vi "Min_Max_Entry.vi"() -> ()   [LabVIEW 2019]
uses:
  Global Variables/Global_Variables.vi
panel:
  in  "Cancel":bool
  in  "Accept":bool
  in  "Value":dbl
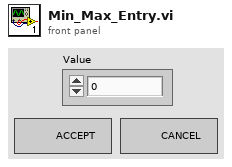
[diagram p1: front panel]
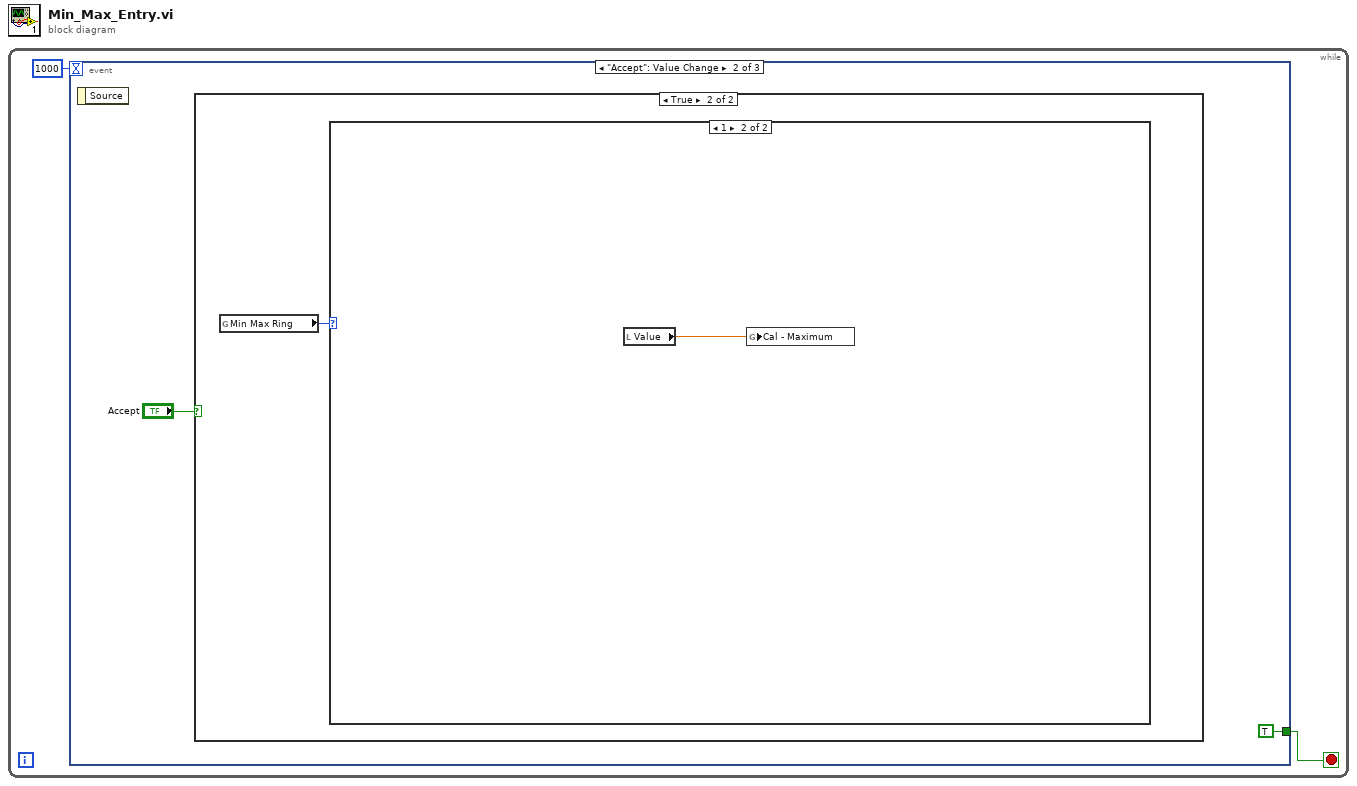
[diagram p0: block diagram]
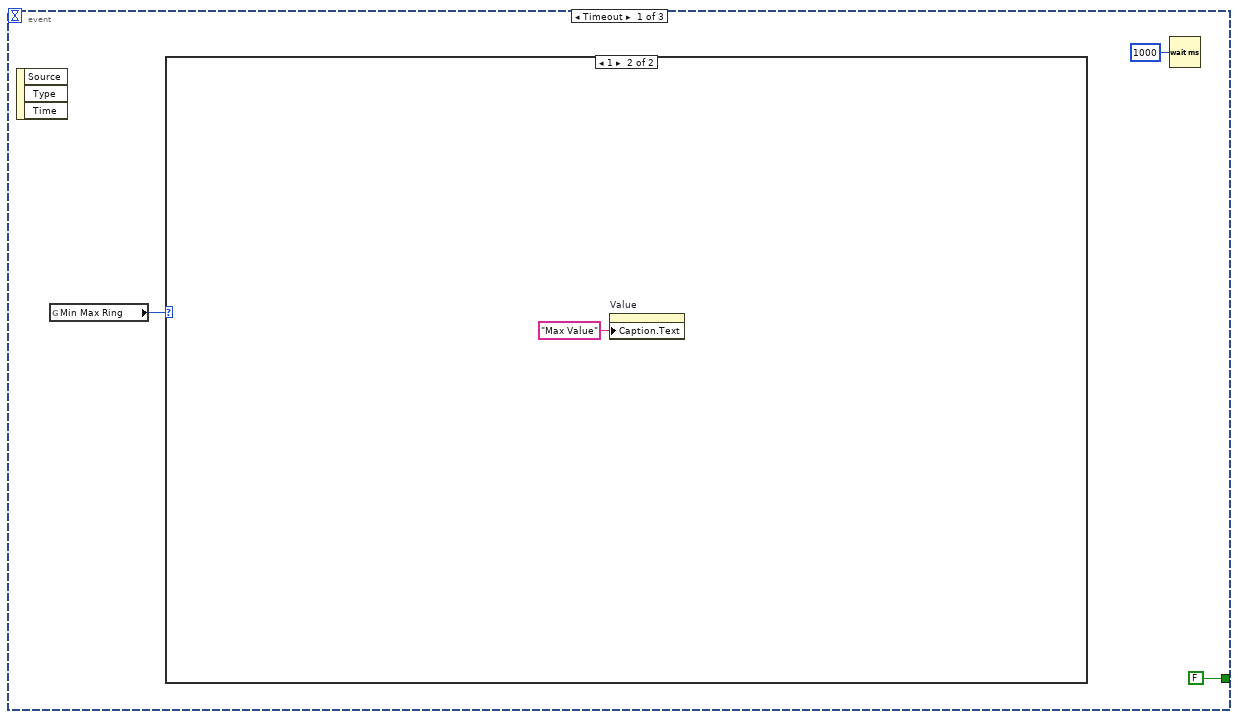
[diagram p2: hidden frame]
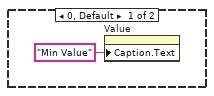
[diagram p3: hidden frame]
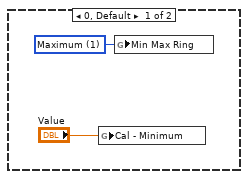
[diagram p5: hidden frame]
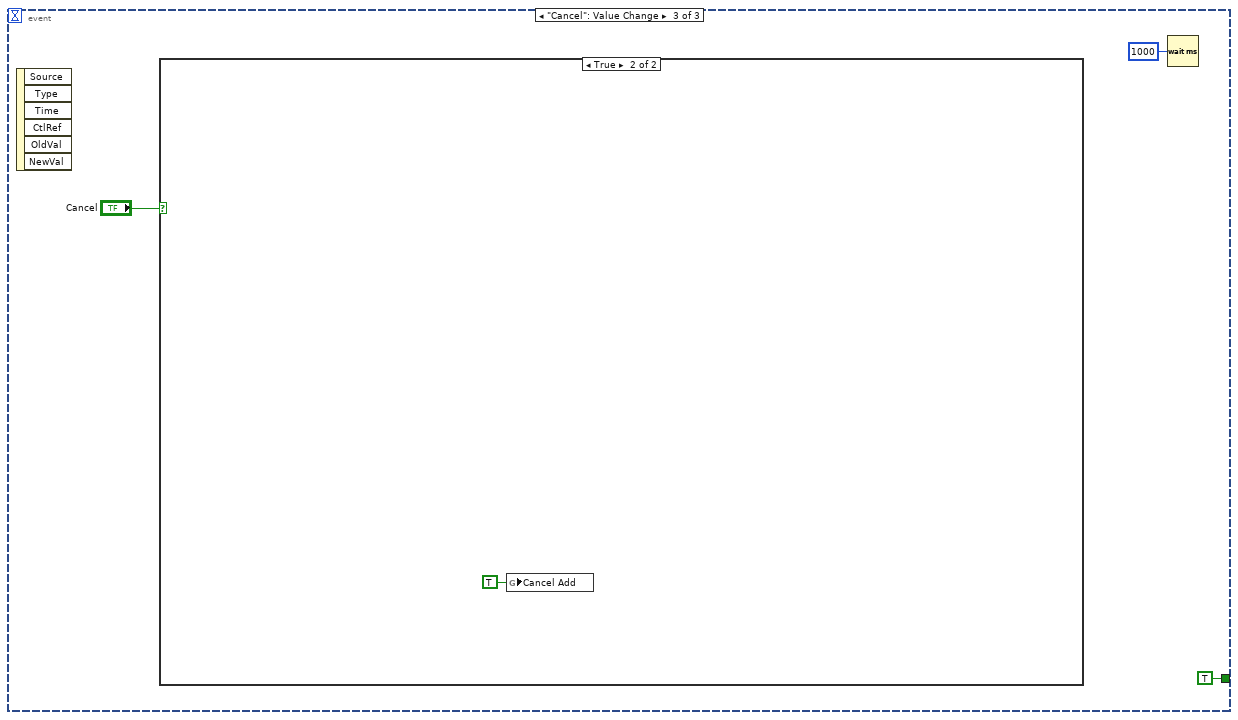
[diagram p6: hidden frame]
diagram:
  n1 = while {
    stop <- w1 stop-if-true
    n2 = event shown="[1] \"Accept\": Value Change" {
      selector: _ -> [_ _ _]
      dyn-events: _ -> [_ _ _]
      timeout: 1000 -> [_ _ _]
      tunnel: [FALSE TRUE TRUE] -> w1
      event Timeout {
        n3 = event-data() -> ()  [unwired: 1 in, 3 out]
        n4 = global read "Global_Variables.vi" "Min Max Ring"() -> (w3:u16)
        n5 = case shown="1" w3 {
          frame 0, Default {
            n6 = property on="Value" class="DigNum (strict)"("Caption.Text"="Min Value") -> ()  [unwired: 2 in, 2 out]
          }
          frame 1 {
            n7 = property on="Value" class="DigNum (strict)"("Caption.Text"="Max Value") -> ()  [unwired: 2 in, 2 out]
          }
        }
        n8 = Wait (ms)(milliseconds to wait=u32 1000) -> ()  [unwired: 1 out]
      }
      event "Accept": Value Change {
        n9 = event-data() -> ()  [unwired: 1 in, 1 out]
        n10 = case shown="True" "Accept" {
          frame False {
          }
          frame True {
            n11 = global read "Global_Variables.vi" "Min Max Ring"() -> (w10:u16)
            n12 = case shown="1" w10 {
              frame 0, Default {
                w11 = u16 1 items=["Minimum", "Maximum"] ("Min Max Ring")
                n13 = global write "Global_Variables.vi" "Cal - Minimum"("Value") -> ()
                n14 = global write "Global_Variables.vi" "Min Max Ring"(w11) -> ()
              }
              frame 1 {
                n15 = local read "Value"() -> (w13:dbl)
                n16 = global write "Global_Variables.vi" "Cal - Maximum"(w13) -> ()
              }
            }
          }
        }
      }
      event "Cancel": Value Change {
        n17 = event-data() -> ()  [unwired: 1 in, 6 out]
        n18 = case shown="True" "Cancel" {
          frame False {
          }
          frame True {
            n19 = global write "Global_Variables.vi" "Cancel Add"(TRUE ("Cancel Add")) -> ()
          }
        }
        n20 = Wait (ms)(milliseconds to wait=u32 1000) -> ()  [unwired: 1 out]
      }
    }
  }
